vi "To JSON.vi"(8 "error in":errorcluster, 10 "JSON Config":path, 11 "IConfigure in":refnum<class "Configuration Base.lvclass">) -> (0 "error out":errorcluster, 3 "IConfigure out":refnum<class "Configuration Base.lvclass">)   [LabVIEW 2023, in "HAL.lvlib" / "Configuration Base.lvclass"]
uses:
  Configuration Base.lvclass
  Configuration Base.lvclass/Configuration Base.ctl
  <vilib>/JDP Science/JSONtext/Config Files/Config File.lvclass
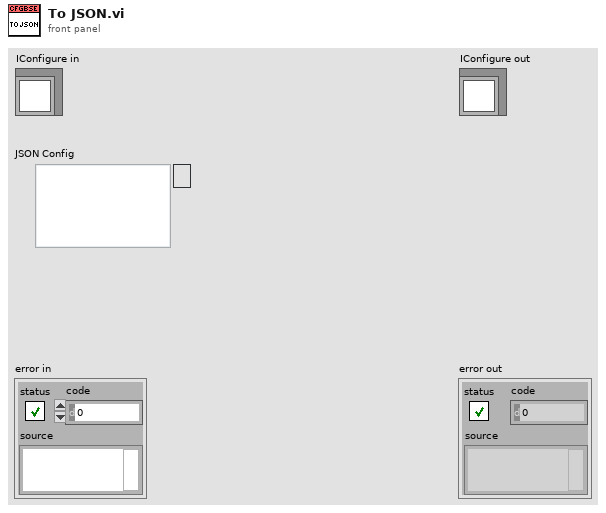
[diagram p1: front panel]
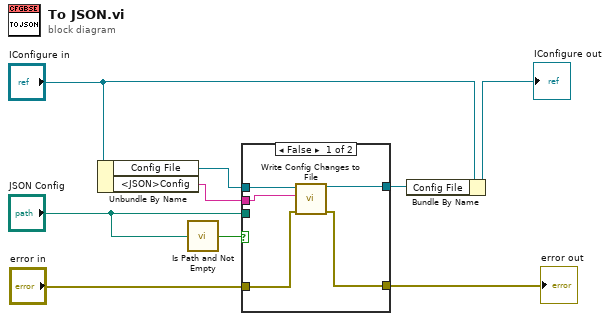
[diagram p0: block diagram]
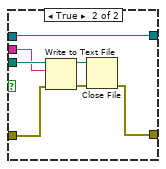
[diagram p2: hidden frame]
diagram:
  n1 = Unbundle By Name("IConfigure in") -> ("Config File"=w6:refnum<class "Config File.lvclass">, "<JSON>Config"=w5:string)
  n2 = call <vilib>:"Is Path and Not Empty.vi"("path"="JSON Config") -> ("Is Path and Not Empty?"=w8:bool)  [unwired: 4 in]
  n3 = case shown="False" w8 {
    tunnel: "JSON Config" -> [_ w21]
    tunnel: w6 -> [w14 w19]
    tunnel: [w10 w19] -> w1
    tunnel: w5 -> [w13 w20]
    tunnel: "error in" -> [w12 w15]
    tunnel: [w11 w16] -> w3
    frame False {
      n4 = call <vilib>:"Write Config Changes to File.vi"("error in (no error)"=w12, "New Config"=w13, "Config File in"=w14) -> ("error out"=w11:errorcluster, "Config File"=w10:refnum<class "Config File.lvclass">)  [unwired: 5 in, 2 out]
    }
    frame True {
      n5 = Write to Text File(file (use dialog)=w21, text=w20, error in=w15) -> (refnum out=w18:refnum<file>, error out=w17:errorcluster)  [unwired: 1 in, 1 out]
      n6 = Close File(refnum=w18, error in=w17) -> (error out=w16:errorcluster)  [unwired: 1 out]
    }
  }
  "error out" <- w3
  n7 = Bundle By Name(cluster="IConfigure in", "Config File"=w1) -> (→"IConfigure out":refnum<class "Configuration Base.lvclass">)
